vi "Register MCP Events.vi"(8 "error in":errorcluster, 10 "User Events":T1) -> (0 "error out":errorcluster)   [LabVIEW 2025, in "Scripting Server.lvlib"]
doc: "Registers the MCP user events in the event handling loop\n\n_____\nCreated using DQMH Framework: Event Scripter 7.1.0.1503."
uses:
  Scripting Server.lvlib
  <vilib>/jgoebel/LabVIEW MCP Server SDK/MCP Server.lvlibp/Praesentationen/MCP in LabVIEW/LabVIEW-MCP-Server-Toolkit/src/MCP Server/onRpc.ctl
  <vilib>/jgoebel/LabVIEW MCP Server SDK/MCP Server.lvlibp
  <vilib>/jgoebel/LabVIEW MCP Server SDK/MCP Server.lvlibp/Praesentationen/MCP in LabVIEW/LabVIEW-MCP-Server-Toolkit/src/MCP Server/Output Parameter.ctl
  <vilib>/jgoebel/LabVIEW MCP Server SDK/MCP Server.lvlibp/Praesentationen/MCP in LabVIEW/LabVIEW-MCP-Server-Toolkit/src/MCP Server/Input Parameter.ctl
  <vilib>/jgoebel/LabVIEW MCP Server SDK/MCP Server.lvlibp/Praesentationen/MCP in LabVIEW/LabVIEW-MCP-Server-Toolkit/src/MCP Server/Tool Data.ctl
  <vilib>/jgoebel/LabVIEW MCP Server SDK/MCP Server.lvlibp/Praesentationen/MCP in LabVIEW/LabVIEW-MCP-Server-Toolkit/src/MCP Server/onTool.ctl
  <vilib>/jgoebel/LabVIEW MCP Server SDK/MCP Server.lvlibp/Praesentationen/MCP in LabVIEW/LabVIEW-MCP-Server-Toolkit/src/MCP Server/onNotification.ctl
  <vilib>/jgoebel/LabVIEW MCP Server SDK/MCP Server.lvlibp/Praesentationen/MCP in LabVIEW/LabVIEW-MCP-Server-Toolkit/src/MCP Server/onToolsCall.ctl
  <vilib>/jgoebel/LabVIEW MCP Server SDK/MCP Server.lvlibp/Praesentationen/MCP in LabVIEW/LabVIEW-MCP-Server-Toolkit/src/MCP Server/onToolsList.ctl
  <vilib>/jgoebel/LabVIEW MCP Server SDK/MCP Server.lvlibp/Praesentationen/MCP in LabVIEW/LabVIEW-MCP-Server-Toolkit/src/MCP Server/onConnect.ctl
  <vilib>/jgoebel/LabVIEW MCP Server SDK/MCP Server.lvlibp/Praesentationen/MCP in LabVIEW/LabVIEW-MCP-Server-Toolkit/src/MCP Server/onLog.ctl
  <vilib>/jgoebel/LabVIEW MCP Server SDK/MCP Server.lvlibp/Praesentationen/MCP in LabVIEW/LabVIEW-MCP-Server-Toolkit/src/MCP Server/User Events.ctl
  Register MCP Events Argument--cluster.ctl
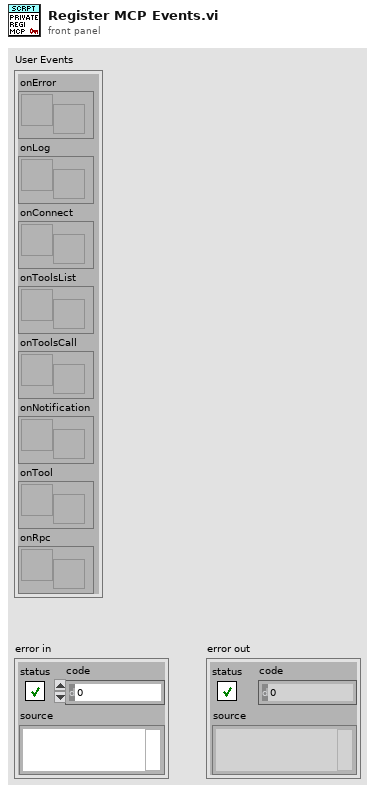
[diagram p1: front panel]
types:
  T1 = typedef "MCP Server.lvlibp/User Events.ctl" = cluster{"onError":refnum<user-event>, "onLog":refnum<user-event>, "onConnect":refnum<user-event>, "onToolsList":refnum<user-event>, "onToolsCall":refnum<user-event>, "onNotification":refnum<user-event>, "onTool":refnum<user-event>, "onRpc":refnum<user-event>}
  T2 = typedef "Scripting Server.lvlib/Register MCP Events Argument--cluster.ctl" = cluster{"User Events":T1}
  T3 = typedef "Scripting Server.lvlib/Request Events--cluster.ctl" = cluster{"Stop Module":refnum<user-event>, "Show Panel":refnum<user-event>, "Hide Panel":refnum<user-event>, "Get Module Execution Status":refnum<user-event>, "Show Diagram":refnum<user-event>, "New VI":refnum<user-event>, "Add Object":refnum<user-event>, "Connect Objects":refnum<user-event>, "Get Object Terminals":refnum<user-event>, "get vi error list":refnum<user-event>, "Cleanup VI":refnum<user-event>, "create_control":refnum<user-event>, "Run VI":refnum<user-event>, "add_to_selection":refnum<user-event>, "clear_selection_list":refnum<user-event>, "remove_from_selection":refnum<user-event>, "enclose_selection":refnum<user-event>, "rename_object":refnum<user-event>, "set_value":refnum<user-event>, "delete_object":refnum<user-event>, "save_vi":refnum<user-event>, "get_structure_diagram":refnum<user-event>, "add_subvi":refnum<user-event>, "connect_to_pane":refnum<user-event>, "get_object_help":refnum<user-event>, "get_loop_conditional_terminal":refnum<user-event>, "show_conditional_terminal":refnum<user-event>, "get_loop_iteration_terminal":refnum<user-event>, "Read Config Data":refnum<user-event>, "get_allowed_paths":refnum<user-event>, "create_project":refnum<user-event>, "Set Allowed Paths":refnum<user-event>, "open_vi":refnum<user-event>, "Private.Register MCP Events":refnum<user-event>}
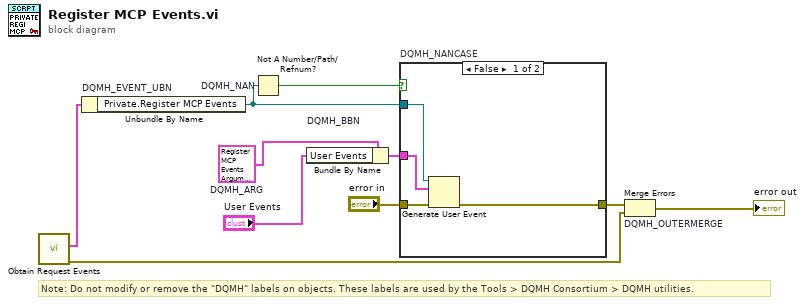
[diagram p0: block diagram]
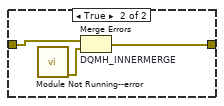
[diagram p2: hidden frame]
diagram:
  w4 = T2 {"User Events"={"onError"=refnum, "onLog"=refnum, "onConnect"=refnum, "onToolsList"=refnum, "onToolsCall"=refnum, "onNotification"=refnum, "onTool"=refnum, "onRpc"=refnum}}  # DQMH_ARG
  # "Note: Do not modify or remove the \"DQMH\" labels on objects. These labels are used by the Tools > DQMH Consortium > DQMH utilities."
  n1 = call "Obtain Request Events.vi"() -> ("error out"=w2:errorcluster, "Scripting Server Request Events"=w1:T3)  [unwired: 10 in]
  n2 = Unbundle By Name "DQMH_EVENT_UBN"(w1) -> ("Private.Register MCP Events"=w6:refnum<user-event>)
  n3 = Not A Number/Path/Refnum? "DQMH_NAN"(number/path/refnum=w6) -> (NaN/Path/Refnum?=w7:bool)
  n4 = Bundle By Name "DQMH_BBN"(cluster=w4, "User Events"="User Events") -> (w8:T2)
  n5 = case "DQMH_NANCASE" shown="False" w7 {
    tunnel: "error in" -> [w14 w17]
    tunnel: [w13 w16] -> w5
    tunnel: w6 -> [w12 _]
    tunnel: w8 -> [w11 _]
    frame False {
      n6 = Generate User Event(user event=w12, event data cluster=w11, error in=w14) -> (error out=w13:errorcluster)  [unwired: 1 in, 1 out]
    }
    frame True {
      n7 = call "Module Not Running--error.vi"() -> ("error out"=w15:errorcluster)  [unwired: 11 in]
      n8 = Merge Errors "DQMH_INNERMERGE"(w17, w15) -> (w16:errorcluster)
    }
  }
  n9 = Merge Errors "DQMH_OUTERMERGE"(w5, w2) -> (→"error out":errorcluster)
